vi "Timer.vi"(8 "error in (no error)":errorcluster, 9 "Stop":bool, 10 "Reset":bool, 11 "Set time":dbl) -> (0 "error out":errorcluster, 2 "Time has Elapsed":bool, 3 "Time left":dbl)   [LabVIEW 2020]
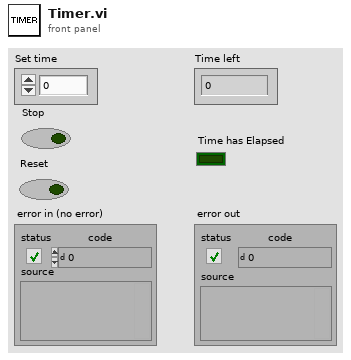
[diagram p1: front panel]
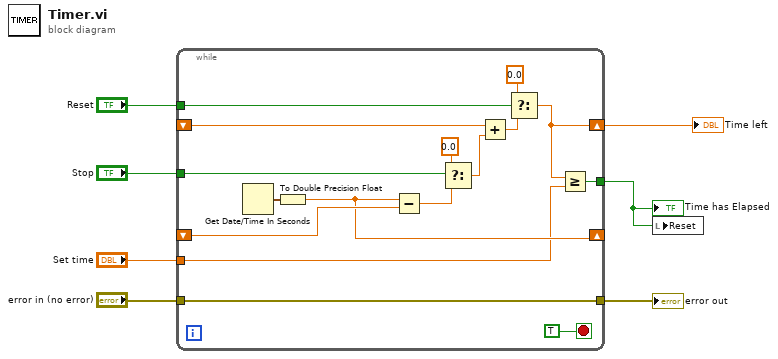
[diagram p0: block diagram]
diagram:
  n1 = while {
    shift-right: [w20] -> _
    shift-left: _ -> [w22]
    tunnel: "Stop" -> [w19]
    tunnel: "Reset" -> [w15]
    shift-right: [w11] -> w1
    shift-left: _ -> [w12]
    tunnel: "Set time" -> [w10]
    tunnel: [w9] -> w5
    tunnel: "error in (no error)" -> [w8]
    tunnel: [w8] -> w3
    stop <- TRUE stop-if-true
    n2 = Get Date/Time In Seconds() -> (seconds since 1Jan1904=w21:timestamp)
    n3 = To Double Precision Float(number=w21) -> (double precision float=w20:dbl)
    n4 = Subtract(x=w20, y=w22) -> (x-y=w18:dbl)
    n5 = Select(t=0.0, s=w19, f=w18) -> (s? t:f=w13:dbl)
    n6 = Add(x=w12, y=w13) -> (x+y=w16:dbl)
    n7 = Select(t=0.0, s=w15, f=w16) -> (s? t:f=w11:dbl)
    n8 = Greater Or Equal?(x=w11, y=w10) -> (x >= y?=w9:bool)
  }
  "error out" <- w3
  "Time left" <- w1
  "Time has Elapsed" <- w5
  n9 = local write "Reset"(w5) -> ()
